vi "ProcessCANRead.vi"(6 "Read_Values in":sgl[](array[numeric]), 8 "error in (no error)":errorcluster, 9 "IDs":sgl[](array[numeric]), 10 "CAN frame":T2 {"type" items=["CAN Data", "CAN Remote"]; "identifier" format="%.0x"}, 11 "ReadFramesInfo":T1(array[cluster])) -> (0 "error out":errorcluster, 2 "ReadFramesSize":i32, 4 "Read_Values out":sgl[](array[numeric]))   [LabVIEW 2016, in "DSI-RT.lvlib"]
uses:
  DSI-RT.lvlib
  <vilib>/RioEmbeddedCAN/RioEmbeddedCAN.llb/CANFrameControl.ctl
  <vilib>/addons/Software Calibration Management/xSCM/SubVIs/Variant Type Index.vi
  <vilib>/addons/Software Calibration Management/xSCM/SubVIs/Variant Element By Index.vi
  <vilib>/addons/Software Calibration Management/xSCM/SubVIs/Variant Element Set.vi
  <vilib>/addons/Software Calibration Management/xSCM/Get/Get Variant.vi
  <vilib>/addons/Software Calibration Management/xSCM/SubVIs/Variant Data Index.vi
  <vilib>/addons/Software Calibration Management/xSCM/Set/Set Variant.vi
  <vilib>/addons/Software Calibration Management/xSCM/SCM-API.lvlib
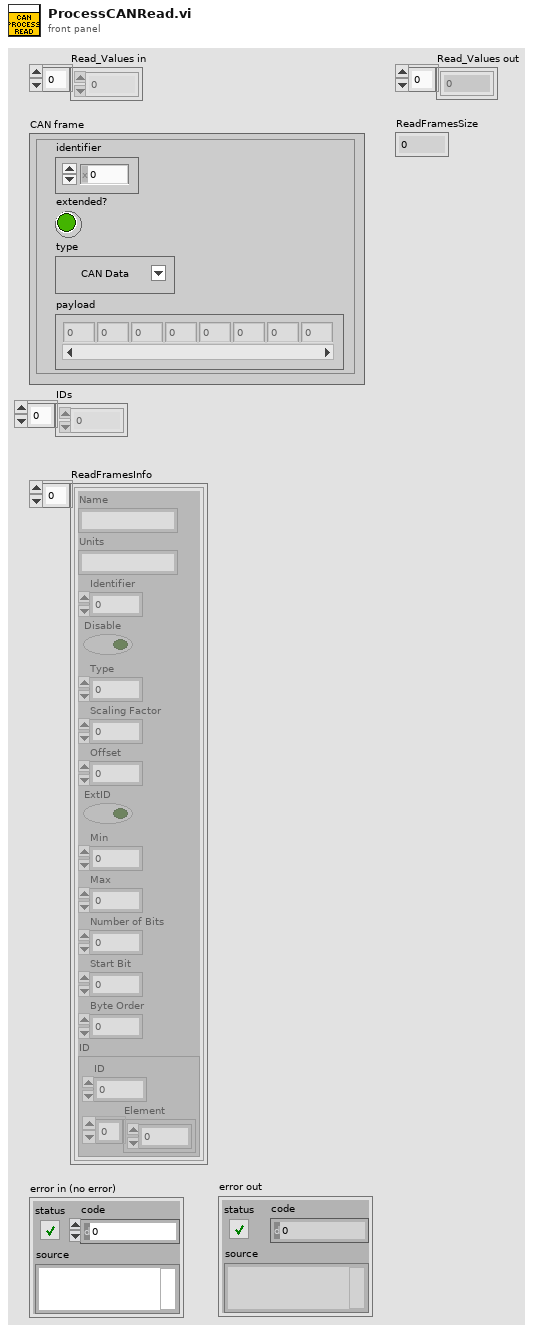
[diagram p1: front panel]
types:
  T1 = cluster{"Name":string, "Units":string, "Identifier":u32, "Disable":bool, "Type":u16, "Scaling Factor":sgl, "Offset":sgl, "ExtID":bool, "Min":sgl, "Max":sgl, "Number of Bits":u8, "Start Bit":u8, "Byte Order":u8, "ID":cluster{"ID":u32, "Element":i32[]}}[]
  T2 = typedef "CANFrameControl.ctl" = cluster{"identifier":u32, "extended?":bool, "type":u8, "payload":u8[]}
  T3 = cluster{"StartBit":u8, "Num Bits":u8, "Byte Order":u8, "Data Type":u8}
  T4 = cluster{"ScalingFactor":sgl, "Offset":sgl, "Maximum":sgl, "Minimum":sgl}
  T5 = cluster{"Name":string, "Units":string, "Identifier":u32, "Disable":bool, "Type":u16, "Scaling Factor":sgl, "Offset":sgl, "ExtID":bool, "Min":sgl, "Max":sgl, "Number of Bits":u8, "Start Bit":u8, "Byte Order":u8, "ID":cluster{"ID":u32, "Element":i32[]}}
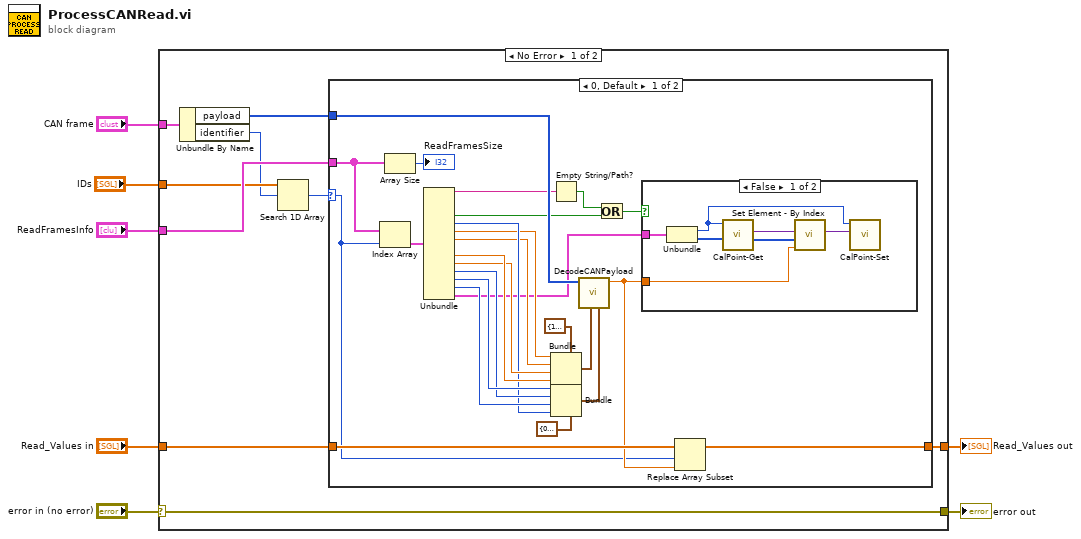
[diagram p0: block diagram]
diagram:
  n1 = case shown="No Error" "error in (no error)" {
    selector: "error in (no error)" -> [w12 w49]
    tunnel: "Read_Values in" -> [w14 w50]
    tunnel: [w13 w50] -> w7
    tunnel: "ReadFramesInfo" -> [w11 _]
    tunnel: "CAN frame" -> [w15 _]
    tunnel: [w12 w49] -> w2
    tunnel: "IDs" -> [w10 _]
    frame No Error {
      n2 = Unbundle By Name(w15) -> ("payload"=w16:u8[], "identifier"=w9:u32)
      n3 = Search 1D Array(1D array=w10, element=w9) -> (index of element=w8:i32)  [unwired: 1 in]
      n4 = case shown="0, Default" w8 {
        selector: w8 -> [w17 _]
        tunnel: w16 -> [w41 _]
        tunnel: w14 -> [w40 w48]
        tunnel: [w39 w48] -> w13
        tunnel: w11 -> [w37 _]
        frame 0, Default {
          n5 = Index Array(array=w37, index=w17) -> (element=w30:T5)
          n6 = Array Size(array=w37) -> (size(s)=→"ReadFramesSize":i32)
          n7 = Unbundle(w30) -> ("Name"=w29:string, "Disable"=w27:bool, "Type"=w21:u16, "Scaling Factor"=w20:sgl, "Offset"=w19:sgl, "Min"=w23:sgl, "Max"=w22:sgl, "Number of Bits"=w24:u8, "Start Bit"=w25:u8, "Byte Order"=w26:u8, "ID"=w18:cluster{"ID":u32, "Element":i32[]})  [unwired: 3 out]
          n8 = Empty String/Path?(string/path=w29) -> (empty?=w28:bool)
          n9 = Bundle(cluster=T4 {"ScalingFactor"=1.0, "Offset"=0.0, "Maximum"=1.0, "Minimum"=0.0} ("DataFormat"), "ScalingFactor"=w20, "Offset"=w19, "Maximum"=w22, "Minimum"=w23) -> (w32:T4)
          n10 = Bundle(cluster=T3 {"StartBit"=0, "Num Bits"=0, "Byte Order"=1, "Data Type"=1} ("ByteFormat"), "StartBit"=w25, "Num Bits"=w24, "Byte Order"=w26, "Data Type"=w21) -> (w33:T3)
          n11 = call "DecodeCANPayload.vi"("ByteFormat"=w33, "DataFormat"=w32, "payload"=w41) -> ("Value"=w36:sgl)  [unwired: 8 in]
          n12 = Or(x=w28, y=w27) -> (x .or. y?=w31:bool)
          n13 = case shown="False" w31 {
            tunnel: w36 -> [w43 _]
            tunnel: w18 -> [w42 _]
            frame False {
              n14 = Unbundle(w42) -> ("ID"=w47:u32, "Element"=w45:i32[])
              n15 = call-poly <vilib>:"CalPoint-Get.vi"("ID"=w47) -> ("Data"=w44:variant)  [unwired: 10 in]
              n16 = call <vilib>:"Set Element - By Index.vi"("Element"=w43, "Elements"=w45, "Variant"=w44) -> ("Variant"=w46:variant)  [unwired: 8 in]
              n17 = call-poly <vilib>:"CalPoint-Set.vi"("Data"=w46, "ID"=w47) -> ()  [unwired: 10 in]
            }
            frame True {
            }
          }
          n18 = Replace Array Subset(array=w40, new element=w36, index=w17) -> (w39:sgl[])
        }
        frame -1 {
        }
      }
    }
    frame Error {
    }
  }
  "Read_Values out" <- w7
  "error out" <- w2
